vi "Exemple2.vi"() -> ()   [LabVIEW 2018]
panel:
  out "Réponse":string
  in  "b":dbl
  in  "a":dbl
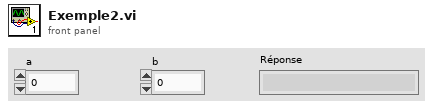
[diagram p1: front panel]
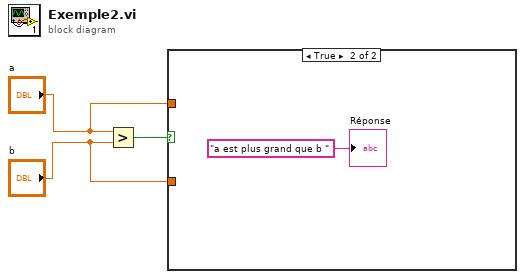
[diagram p0: block diagram]
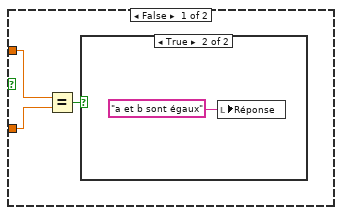
[diagram p2: hidden frame]
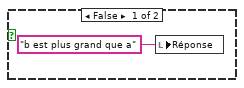
[diagram p3: hidden frame]
diagram:
  n1 = Greater?(x="a", y="b") -> (0:w3:bool)
  n2 = case shown="True" w3 {
    tunnel: "a" -> [w5 _]
    tunnel: "b" -> [w4 _]
    frame False {
      n3 = Equal?(x=w5, y=w4) -> (x = y?=w6:bool)
      n4 = case shown="True" w6 {
        frame False {
          n5 = local write "Réponse"("b est plus grand que a" ("Réponse")) -> ()
        }
        frame True {
          n6 = local write "Réponse"("a et b sont égaux" ("Réponse")) -> ()
        }
      }
    }
    frame True {
      "Réponse" <- "a est plus grand que b "
    }
  }
